vi "Serial Test.vi"() -> ()   [LabVIEW 2014]
uses:
  <vilib>/Instr/_visa.llb/VISA Configure Serial Port (Instr).vi
panel:
  in  "Write?":bool
  in  "write buffer":string
  out "empty?":bool
  in  "timeout (10sec)":u32=10000
  in  "termination char\n(0xA = '\\n' = LF)":u8=10 format="%.0x"
  in  "Enable Termination\nChar (T)":bool=TRUE
  in  "flow control (0:none)":u16(ring) items=["None", "XON/XOFF", "RTS/CTS", "XON/XOFF & RTS/CTS", "DTR/DSR", "XON/XOFF & DTR/DSR"]
  in  "stop bits (10: 1 bit)":u16(ring)=10 items=["1.0"=10, "1.5"=15, "2.0"=20]
  in  "parity (0:none)":enum16{"None", "Odd", "Even", "Mark", "Space"}(ring)
  in  "data bits (8)":u16=8 min=5 max=8 step=1
  out "Bytes at port":u32
  in  "Stop":bool
  out "Bytes read":u32
  out "Bytes written":u32
  out "Read Buffer":string
  in  "baud rate (19200)":u32=19200
  in  "VISA resource name":refnum<visa-resource-name>="COM4"
  # "Serial Settings"
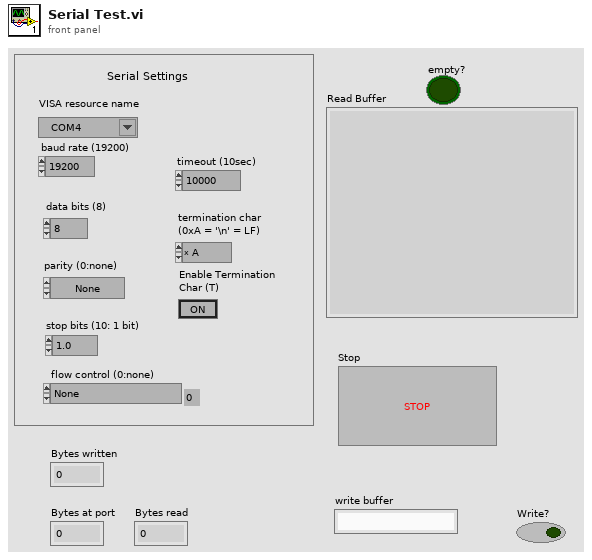
[diagram p1: front panel]
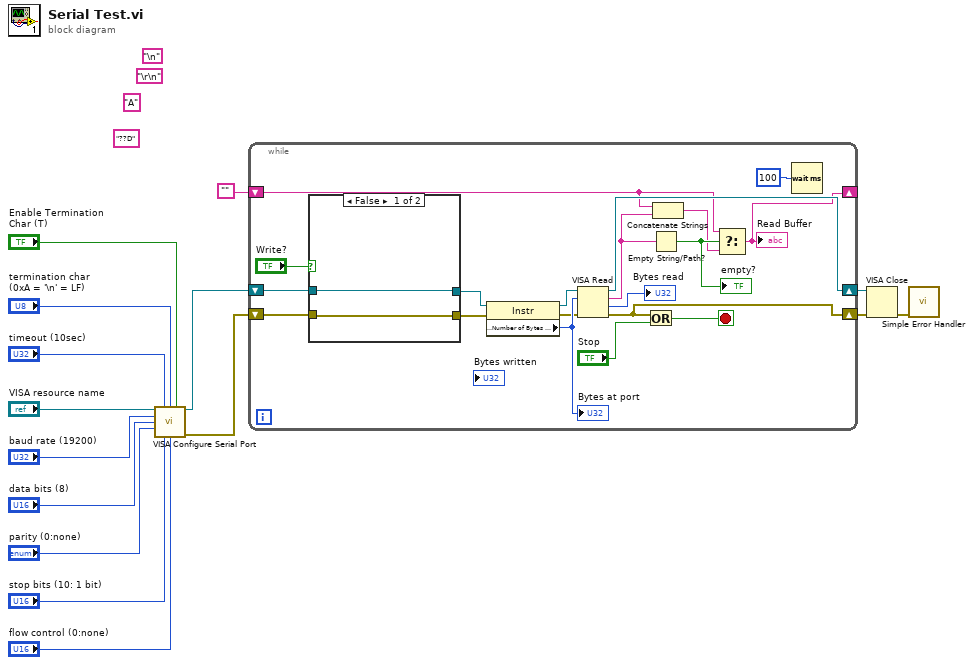
[diagram p0: block diagram]
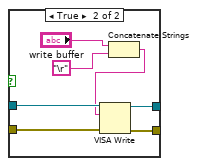
[diagram p2: hidden frame]
diagram:
  (unwired) "??D" ("write buffer")
  (unwired) "\r\n"
  (unwired) "\n"
  (unwired) "A" ("write buffer")
  n1 = call-poly "VISA Configure Serial Port"("VISA resource name"="VISA resource name", "timeout (10sec)"="timeout (10sec)", "termination char\n(0xA = '\\n' = LF)"="termination char\n(0xA = '\\n' = LF)", "Enable Termination\nChar (T)"="Enable Termination\nChar (T)", "baud rate (9600)"="baud rate (19200)", "data bits (8)"="data bits (8)", "parity (0:none)"="parity (0:none)", "stop bits (10: 1 bit)"="stop bits (10: 1 bit)", "flow control (0:none)"="flow control (0:none)") -> ("VISA resource name out"=w1:refnum<visa-resource-name>, "error out"=w2:errorcluster)  [unwired: 5 in]
  n2 = while {
    shift-right: [w22] -> _
    shift-left: "" -> [w25]
    shift-right: [w31] -> w13
    shift-left: w1 -> [w20]
    shift-right: [w21] -> w10
    shift-left: w2 -> [w19]
    stop <- w28 stop-if-true
    n3 = case shown="False" "Write?" {
      tunnel: w20 -> [w36 w43]
      tunnel: w19 -> [w35 w42]
      tunnel: [w35 w41] -> w18
      tunnel: [w36 w40] -> w17
      frame False {
      }
      frame True {
        n4 = Concatenate Strings("write buffer", "\r") -> (w37:string)
        n5 = VISA Write(VISA resource name=w43, write buffer=w37, error in (no error)=w42) -> (VISA resource name out=w40:refnum<visa-resource-name>, error out=w41:errorcluster)  [unwired: 1 out]
      }
    }
    n6 = property class="Instr"(reference=w17, error in=w18) -> (reference out=w33:refnum<visa-resource-name>, error out=w32:errorcluster, "Serial Settings:Number of Bytes at Serial Port"=w34:u32)
    "Bytes at port" <- w34
    n7 = VISA Read(VISA resource name=w33, byte count=w34, error in (no error)=w32) -> (VISA resource name out=w31:refnum<visa-resource-name>, read buffer=w24:string, return count=→"Bytes read":u32, error out=w21:errorcluster)
    n8 = Or(x=w21, y="Stop") -> (x .or. y?=w28:bool)
    n9 = Empty String/Path?(string/path=w24) -> (empty?=w26:bool)
    "empty?" <- w26
    n10 = Concatenate Strings(w25, w24) -> (w23:string)
    n11 = Select(t=w25, s=w26, f=w23) -> (s? t:f=w22:string)
    "Read Buffer" <- w22
    n12 = Wait (ms)(milliseconds to wait=u32 100) -> ()  [unwired: 1 out]
  }
  n13 = VISA Close(VISA resource name=w13, error in (no error)=w10) -> (error out=w12:errorcluster)
  n14 = call <vilib>:"Simple Error Handler.vi"("error in (no error)"=w12) -> ()  [unwired: 4 in, 5 out]
